vi "SP Perform Limit Testing.vi"(4 "Generate Plot Output? (f)":bool, 7 "Filled Limits? (f)":bool, 8 "error in (no error)":errorcluster, 9 "LLimits":cluster{"x0":dbl, "dx":dbl, "Y":dbl[]}[](array[cluster]), 10 "ULimits":cluster{"x0":dbl, "dx":dbl, "Y":dbl[]}[](array[cluster]), 11 "Data":cluster{"x0":dbl, "dx":dbl, "Y":dbl[]}) -> (0 "error out":errorcluster, 1 "Lower Pass?":bool, 2 "Upper Pass?":bool, 3 "Plot Output":cluster{"x0":dbl, "dx":dbl, "Y":dbl[]}[](array[cluster]) {"Y" format="%.2p"; "dx" format="%.2p"; "x0" format="%.2p"}, 5 "Failures":cluster{"x values":dbl[], "y values":dbl[]}[](array[cluster]))   [LabVIEW 2011]
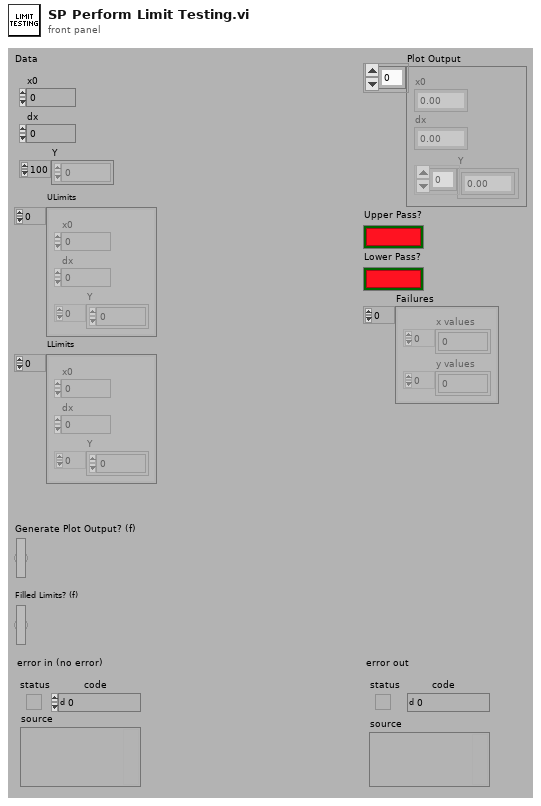
[diagram p1: front panel]
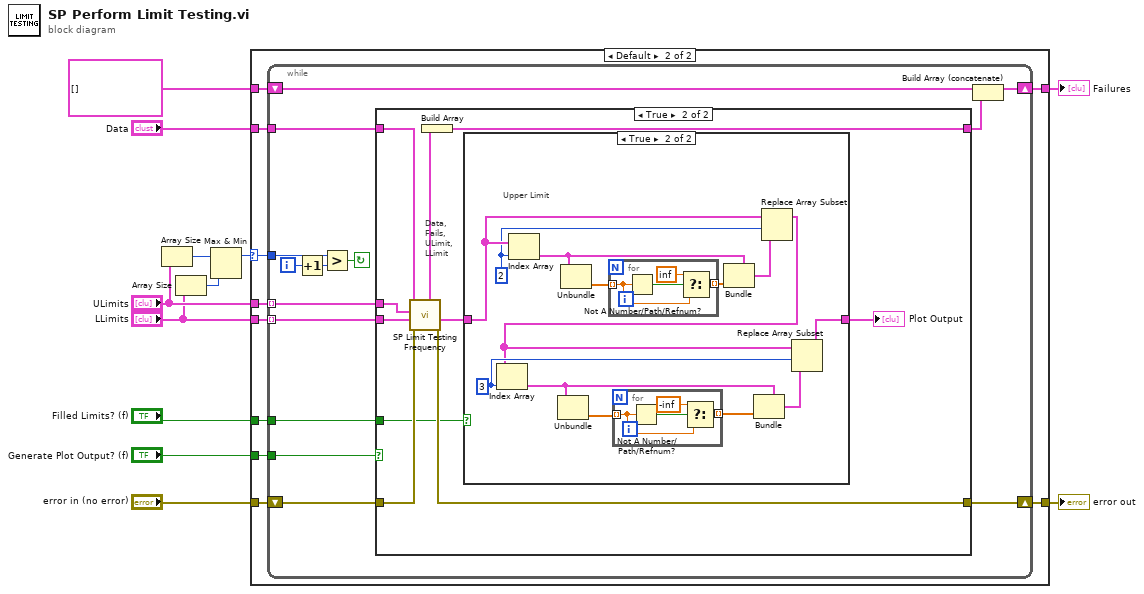
[diagram p0: block diagram]
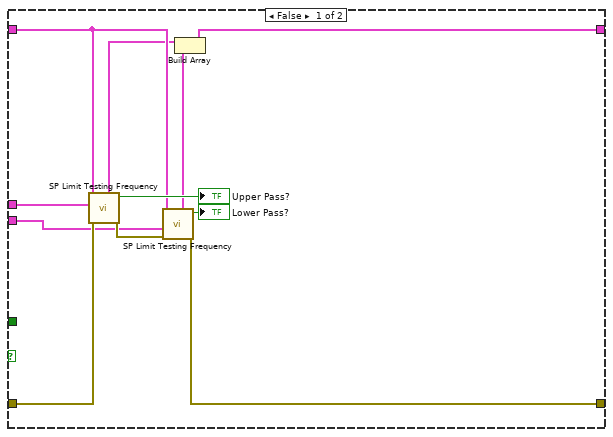
[diagram p3: hidden frame]
diagram:
  n1 = Array Size(array="ULimits") -> (size(s)=w2:i32)
  n2 = Array Size(array="LLimits") -> (size(s)=w3:i32)
  n3 = Max & Min(x=w2, y=w3) -> (max(x,y)=w1:i32)  [unwired: 1 out]
  n4 = case shown="Default" w1 {
    selector: w1 -> [_ w15]
    tunnel: "error in (no error)" -> [w14 w24]
    tunnel: [w14 w23] -> w11
    tunnel: "Generate Plot Output? (f)" -> [_ w22]
    tunnel: "Data" -> [_ w21]
    tunnel: "Filled Limits? (f)" -> [_ w20]
    tunnel: [w13 w19] -> w7
    tunnel: cluster{"x values":dbl[], "y values":dbl[]}[] [] ("Failures") -> [w13 w18]
    tunnel: "ULimits" -> [_ w17]
    tunnel: "LLimits" -> [_ w16]
    frame 0 {
    }
    frame Default {
      n5 = while {
        tunnel: w17 -> [w25] mode=indexing
        tunnel: w16 -> [w26] mode=indexing
        tunnel: w22 -> [w36]
        tunnel: w21 -> [w35]
        tunnel: w20 -> [w34]
        shift-right: [w32] -> w19
        shift-left: w18 -> [w33]
        shift-right: [w37] -> w23
        shift-left: w24 -> [w38]
        tunnel: w15 -> [w30]
        i -> [w27]
        stop <- w28 continue-if-true
        n6 = Increment(x=w27) -> (x+1=w29:i32)
        n7 = Greater?(x=w30, y=w29) -> (0:w28:bool)
        n8 = case shown="True" w36 {
          tunnel: w25 -> [w48 w59]
          tunnel: w26 -> [w43 w58]
          tunnel: w38 -> [w49 w57]
          tunnel: [w44 w56] -> w37
          tunnel: w35 -> [w42 w55]
          tunnel: w34 -> [_ w52]
          tunnel: [w39 w50] -> w31
          frame False {
            n9 = call "SP Limit Testing Frequency.vi"("error in"=w49, "upper limit"=w48, "signal in"=w42) -> ("error out"=w46:errorcluster, "test passed?"=→"Upper Pass?":bool, "failures"=w41:cluster{"x values":dbl[], "y values":dbl[]})  [unwired: 2 in, 4 out]
            n10 = call "SP Limit Testing Frequency.vi"("error in"=w46, "lower limit"=w43, "signal in"=w42) -> ("error out"=w44:errorcluster, "test passed?"=→"Lower Pass?":bool, "failures"=w40:cluster{"x values":dbl[], "y values":dbl[]})  [unwired: 2 in, 4 out]
            n11 = Build Array(w41, w40) -> (w39:cluster{"x values":dbl[], "y values":dbl[]}[])
          }
          frame True {
            # "Data,\nFails,\nULimit,\nLLimit"
            n12 = call "SP Limit Testing Frequency.vi"("error in"=w57, "lower limit"=w58, "upper limit"=w59, "signal in"=w55) -> ("error out"=w56:errorcluster, "output values"=w54:cluster{"x0":dbl, "dx":dbl, "Y":dbl[]}[], "failures"=w51:cluster{"x values":dbl[], "y values":dbl[]})  [unwired: 1 in, 4 out]
            n13 = Build Array(w51) -> (w50:cluster{"x values":dbl[], "y values":dbl[]}[])
            n14 = case shown="True" w52 {
              tunnel: w54 -> [w60 w70]
              tunnel: [w60 w61] -> w53
              frame False {
              }
              frame True {
                w63 = 3 ("index")
                w69 = 2 ("index")
                # "Upper Limit"
                n15 = Index Array(array=w70, index=w69) -> (element=w72:cluster{"x0":dbl, "dx":dbl, "Y":dbl[]})
                n16 = Unbundle(w72) -> ("Y"=w73:dbl[])  [unwired: 2 out]
                n17 = for {
                  tunnel: w73 -> [w80] mode=indexing
                  tunnel: [w79] -> w71 mode=indexing
                  n18 = Not A Number/Path/Refnum?(number/path/refnum=w80) -> (NaN/Path/Refnum?=w81:bool)
                  n19 = Select(t=inf, s=w81, f=w80) -> (s? t:f=w79:dbl)
                }
                n20 = Bundle(cluster=w72, "Y"=w71) -> (w68:cluster{"x0":dbl, "dx":dbl, "Y":dbl[]})  [unwired: 2 out]
                n21 = Replace Array Subset(array=w70, new element=w68, index=w69) -> (w62:cluster{"x0":dbl, "dx":dbl, "Y":dbl[]}[])
                n22 = Index Array(array=w62, index=w63) -> (element=w64:cluster{"x0":dbl, "dx":dbl, "Y":dbl[]})
                n23 = Unbundle(w64) -> ("Y"=w66:dbl[])  [unwired: 2 out]
                n24 = for {
                  tunnel: w66 -> [w76] mode=indexing
                  tunnel: [w75] -> w65 mode=indexing
                  n25 = Not A Number/Path/Refnum?(number/path/refnum=w76) -> (NaN/Path/Refnum?=w77:bool)
                  n26 = Select(t=-inf, s=w77, f=w76) -> (s? t:f=w75:dbl)
                }
                n27 = Bundle(cluster=w64, "Y"=w65) -> (w67:cluster{"x0":dbl, "dx":dbl, "Y":dbl[]})  [unwired: 2 out]
                n28 = Replace Array Subset(array=w62, new element=w67, index=w63) -> (w61:cluster{"x0":dbl, "dx":dbl, "Y":dbl[]}[])
              }
            }
            "Plot Output" <- w53
          }
        }
        n29 = Build Array (concatenate)(w33, w31) -> (w32:cluster{"x values":dbl[], "y values":dbl[]}[])
      }
    }
  }
  "error out" <- w11
  "Failures" <- w7
